vi "Process Player 2 Events.vi"(11 "Main Controller Actor in":refnum<class "Main Controller Actor.lvclass">) -> (3 "Main Controller Actor out":refnum<class "Main Controller Actor.lvclass">)   [LabVIEW 2015, in "Main Controller Actor.lvclass"]
uses:
  Main Controller Actor.lvclass
  Controls/Player.ctl
  Globals.vi
  <userlib>/_OpenG.lib/comparison/comparison.llb/Boolean Changed__ogtk.vi
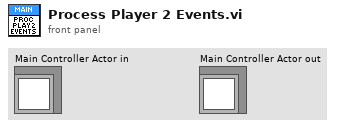
[diagram p1: front panel]
types:
  T1 = typedef "Player.ctl" = enum16{"1", "2"}
  T2 = cluster{"Primary Weapon":bool, "Special Function":bool, "Thrust":bool, "Rotate Clockwise":bool, "Rotate Counter Clockwise":bool}
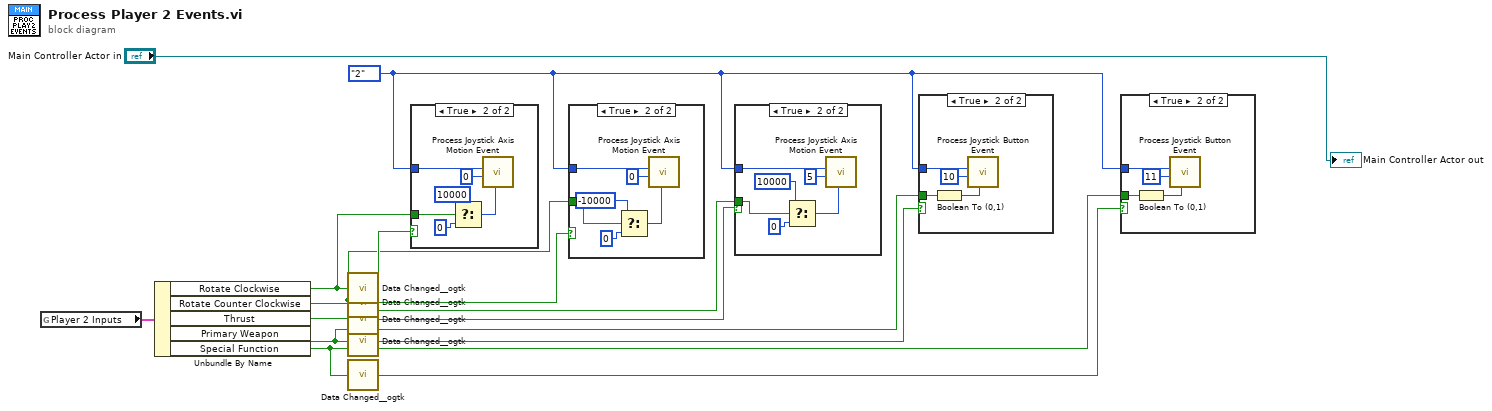
[diagram p0: block diagram]
diagram:
  w2 = Player."2" ("Player")
  n1 = global read "Globals.vi" "Player 2 Inputs"() -> (w13:T2)
  n2 = Unbundle By Name(w13) -> ("Rotate Clockwise"=w4:bool, "Rotate Counter Clockwise"=w3:bool, "Thrust"=w7:bool, "Primary Weapon"=w10:bool, "Special Function"=w11:bool)
  n3 = call-poly <userlib>:"Data Changed__ogtk.vi"("Boolean"=w4) -> ("Changed"=w6:bool)
  n4 = call-poly <userlib>:"Data Changed__ogtk.vi"("Boolean"=w3) -> ("Changed"=w5:bool)
  n5 = call-poly <userlib>:"Data Changed__ogtk.vi"("Boolean"=w7) -> ("Changed"=w8:bool)
  n6 = call-poly <userlib>:"Data Changed__ogtk.vi"("Boolean"=w10) -> ("Changed"=w9:bool)
  n7 = call-poly <userlib>:"Data Changed__ogtk.vi"("Boolean"=w11) -> ("Changed"=w12:bool)
  n8 = case shown="True" w6 {
    tunnel: w2 -> [_ w19]
    tunnel: w4 -> [_ w17]
    frame False {
    }
    frame True {
      n9 = Select(t=i16 10000 ("Value"), s=w17, f=i16 0) -> (s? t:f=w15:i16)
      n10 = call "Process Joystick Axis Motion Event.vi"("Value"=w15, "Axis"=u8 0, "Player"=w19) -> ()  [unwired: 9 in]
    }
  }
  n11 = case shown="True" w5 {
    tunnel: w2 -> [_ w25]
    tunnel: w3 -> [_ w20]
    frame False {
    }
    frame True {
      n12 = Select(t=i16 -10000 ("Value"), s=w20, f=i16 0) -> (s? t:f=w22:i16)
      n13 = call "Process Joystick Axis Motion Event.vi"("Value"=w22, "Axis"=u8 0, "Player"=w25) -> ()  [unwired: 9 in]
    }
  }
  n14 = case shown="True" w8 {
    tunnel: w2 -> [_ w31]
    tunnel: w7 -> [_ w28]
    frame False {
    }
    frame True {
      n15 = Select(t=i16 10000 ("Value"), s=w28, f=i16 0) -> (s? t:f=w27:i16)
      n16 = call "Process Joystick Axis Motion Event.vi"("Value"=w27, "Axis"=u8 5, "Player"=w31) -> ()  [unwired: 9 in]
    }
  }
  n17 = case shown="True" w9 {
    tunnel: w2 -> [_ w35]
    tunnel: w10 -> [_ w33]
    frame False {
    }
    frame True {
      n18 = Boolean To (0,1)(Boolean=w33) -> (0, 1=w32:i16)
      n19 = call "Process Joystick Button Event.vi"("State"=w32, "Button"=u8 10, "Player"=w35) -> ()  [unwired: 9 in]
    }
  }
  n20 = case shown="True" w12 {
    tunnel: w2 -> [_ w39]
    tunnel: w11 -> [_ w37]
    frame False {
    }
    frame True {
      n21 = Boolean To (0,1)(Boolean=w37) -> (0, 1=w36:i16)
      n22 = call "Process Joystick Button Event.vi"("State"=w36, "Button"=u8 11, "Player"=w39) -> ()  [unwired: 9 in]
    }
  }
  "Main Controller Actor out" <- "Main Controller Actor in"
